vi "WorkingDialog.vi"(10 "StopQueue":refnum<queue>, 11 "Text":string) -> ()   [LabVIEW 2020, in "DependencyChecker.lvlib"]
uses:
  <resource>/Framework/Providers/Open_GDS/DependencyViewer/DependencyChecker/DependencyChecker.lvlib
panel:
  out "Time":dbl format="%.1f"
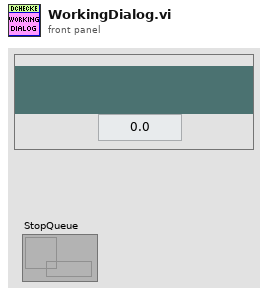
[diagram p1: front panel]
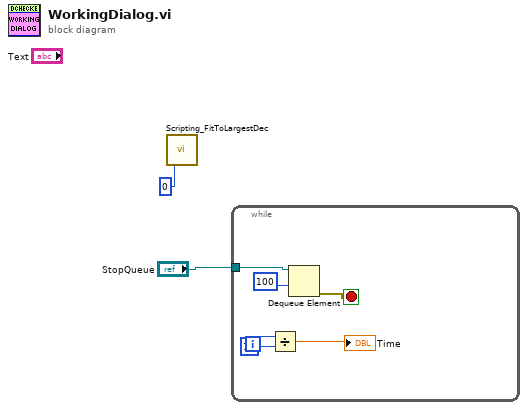
[diagram p0: block diagram]
diagram:
  n1 = call <resource>:"Scripting_FitToLargestDec.vi"("border spacing (2 px)"=0) -> ()  [unwired: 5 in, 2 out]
  n2 = while {
    tunnel: "StopQueue" -> [w7]
    i -> [w6]
    stop <- w3 stop-if-true
    n3 = Divide(x=w6, y=10) -> (x/y=→"Time":dbl)
    n4 = Dequeue Element(queue=w7, timeout in ms (-1)=u32 100 ("milliseconds to wait")) -> (error out=w3:errorcluster)  [unwired: 1 in, 3 out]
  }
